vi "Run.vi"(0 "reg in":refnum<class "bronkhorst_reg_1.lvclass">, 1 "XB24 (F)":bool, 5 "SP":dbl caption="setpoint" step=0.01 format="%.2f", 7 "PV":dbl step=0.01 format="%.2f", 9 "PV_State":T5, 11 "error in (no error)":errorcluster, 12 "Y_in":dbl step=0.01 format="%.2f", 13 "Y_State":T5) -> (4 "reg out":refnum<class "bronkhorst_reg_1.lvclass">, 6 "Y_out":dbl format="%.2f", 8 "T":u32, 10 "End":bool, 15 "error out":errorcluster)   [LabVIEW 2019, in "bronkhorst_reg_1.lvclass"]
uses:
  bronkhorst_reg_1.lvclass
  Inputs/Ctl/Parameter State short.ctl
  ctl/Y_Lim_State.ctl
  ctl/ZY_control_short.ctl
  ctl/Z_State.ctl
  ctl/Y_state.ctl
  bronkhorst_reg_1.lvclass/bronkhorst_reg_1.ctl
  Inputs/Ctl/Sensor state.ctl
  Inputs/Ctl/Sensor alarm.ctl
  ctl/control param simple.ctl
  PID/PID Output Rate Limiter Ext.vi
  PID/PID Timing Estimation Ext.vi
  control.lvlib
  Inputs/Inputs.lvlib
panel:
  out "ZY_control":T1={"Start"=FALSE, "Z_HSw"=0, "Z_HSetState"=enum."on", "Y_HSw"=0, "Y_HSetState"=enum."hand", "SP"=0.0, "Y_H"=0.0, "Reset_ALR"=FALSE} {"Y_H" step=1.0; "SP" step=0.01 format="%.2f"}
  out "SpLim_State":T4=enum."increase"
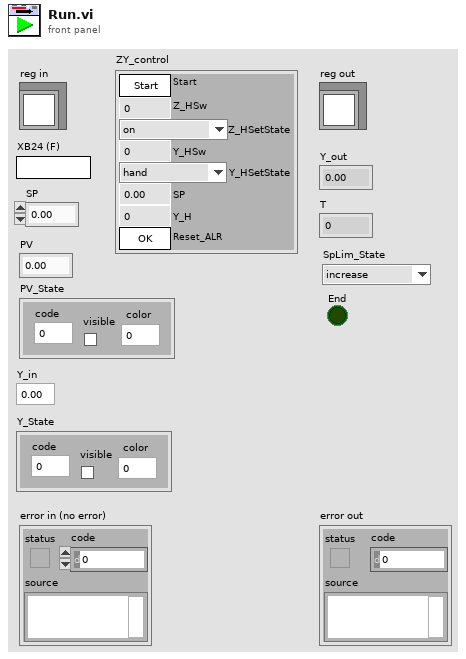
[diagram p1: front panel]
types:
  T1 = typedef "control.lvlib/ZY_control_short.ctl" = cluster{"Start":bool, "Z_HSw":u32, "Z_HSetState":T2, "Y_HSw":u32, "Y_HSetState":T3, "SP":dbl, "Y_H":dbl, "Reset_ALR":bool}
  T2 = typedef "control.lvlib/Z_State.ctl" = enum8{"initialization", "alarm", "disabled", "not ready", "stop ready", "reserv", "switched off", "reserv2", "switched on", "check", "on min", "decrease out", "on", "increase out", "on max"}
  T3 = typedef "control.lvlib/Y_state.ctl" = enum8{"initialize", "alarm", "min", "stop", "hand", "auto", "max"}
  T4 = typedef "control.lvlib/Y_Lim_State.ctl" = enum8{"initialization", "alarm", "stop", "decrease", "increase"}
  T5 = typedef "Inputs.lvlib/Parameter State short.ctl" = cluster{"code":i32, "visible":bool, "color":u32}
  T6 = typedef "Inputs.lvlib/Sensor state.ctl" = cluster{"source":string, "color":u32, "visible":bool}[]
  T7 = typedef "Inputs.lvlib/Sensor alarm.ctl" = cluster{"source":string, "color":u32, "visible":bool}[]
  T8 = typedef "control.lvlib/control param simple.ctl" = cluster{"output high":dbl, "alr value":dbl, "output low":dbl, "output time (t)":dbl}
  T9 = cluster{"Y_HSw":u32, "Y_HSetState":T3, "Y_ASetState":T3, "Y_DSetState":T3}
  T10 = typedef "control.lvlib/control param.ctl" = cluster{"proportional gain (Kc)":dbl, "integral time (Ti, s)":dbl, "derivative time (Td, s)":dbl, "output high":dbl, "output high start":dbl, "output high stop":dbl, "alr value":dbl, "output low":dbl, "output rate (EGU/s)":dbl, "setpoint max":dbl, "setpoint rate (EGU/min)":dbl, "stop rate (EGU/min)":dbl}
  T11 = typedef "control.lvlib/Y_source.ctl" = enum8{"initialize", "local disabled", "local hand", "hand", "auto", "dist"}
  T12 = enum8{"alarm", "min", "stop", "hand", "auto", "max"}
  T13 = typedef "control.lvlib/Y_Lim_ext_defs.ctl" = cluster{"reinitialize":bool, "SpLim_State":T4, "output":dbl, "Tick":u32, "output rate":dbl, "Y_Set":dbl, "Y_preSet":dbl}
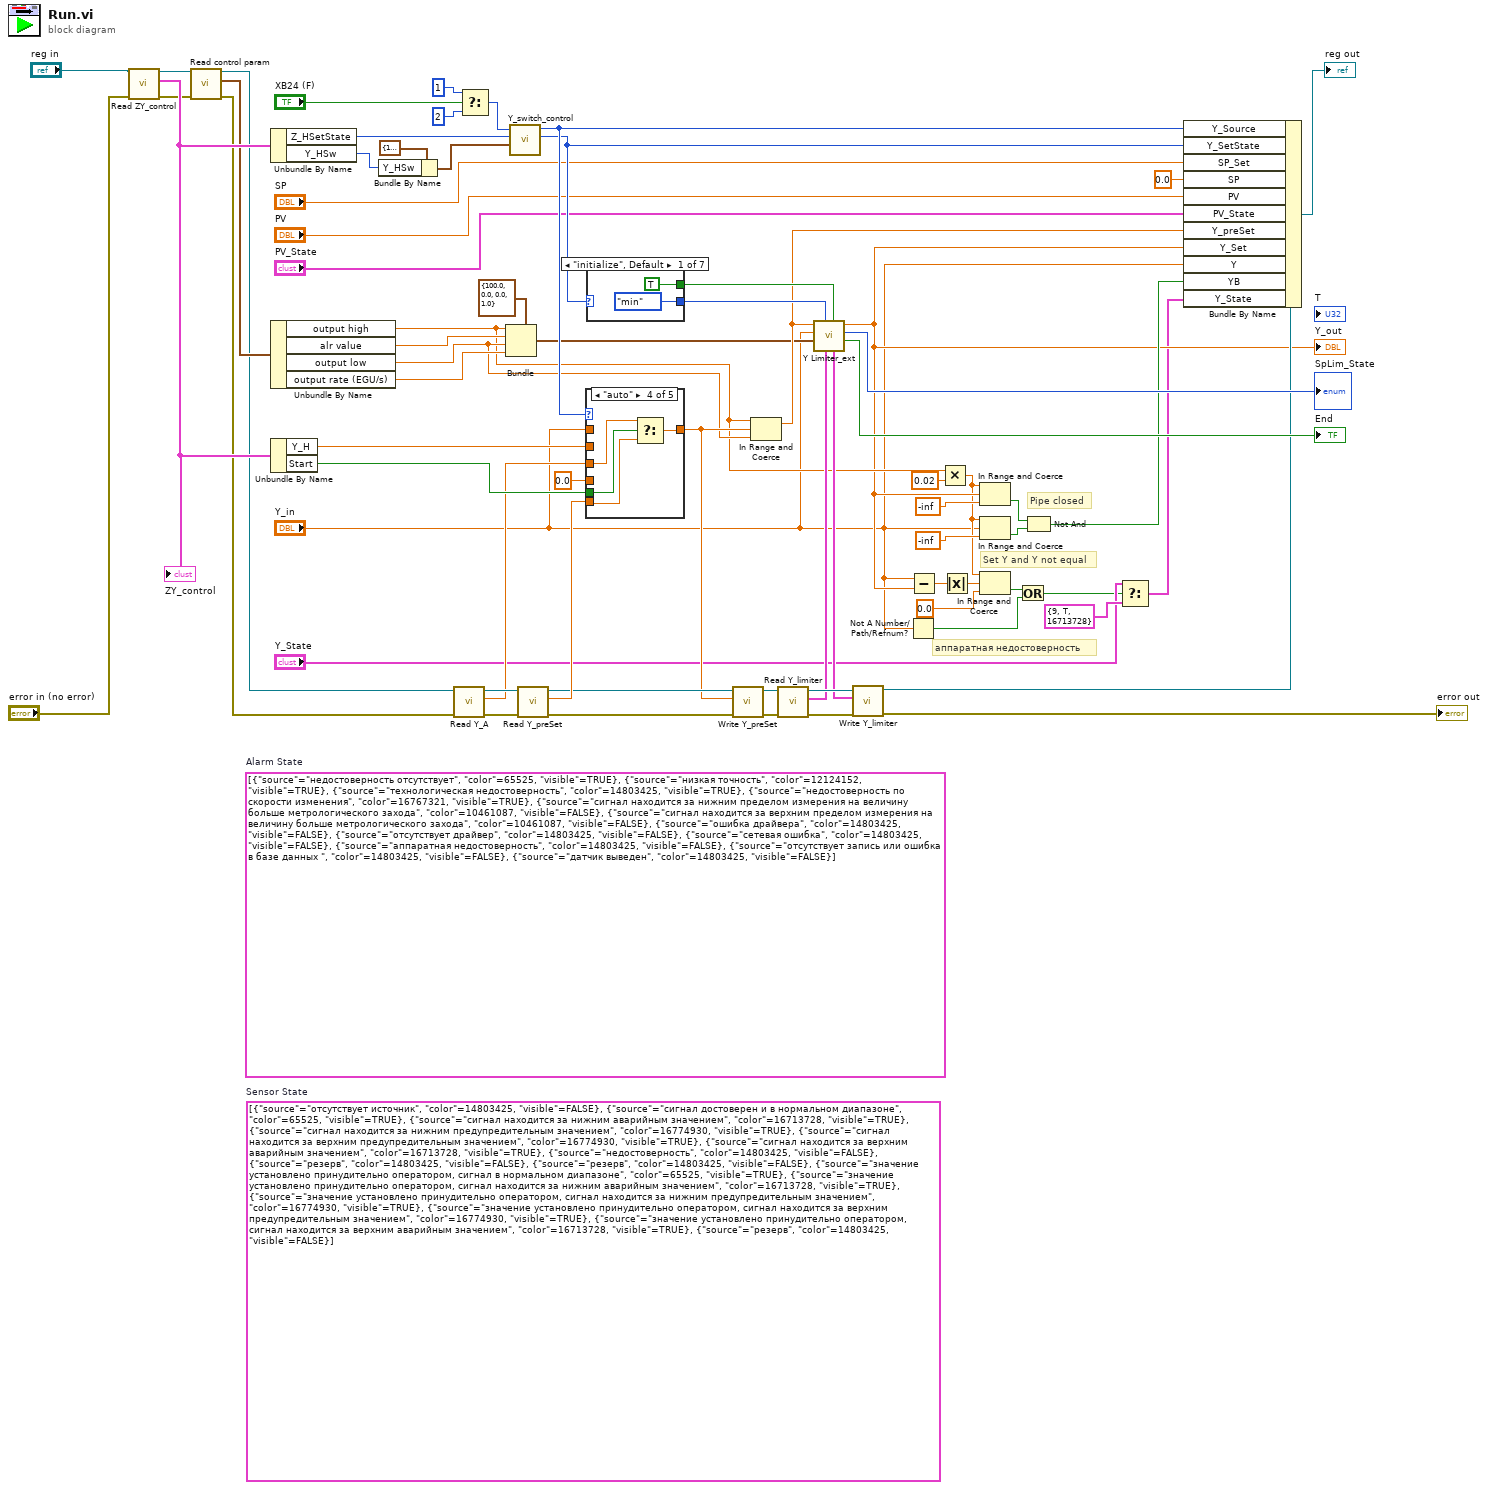
[diagram p0: block diagram]
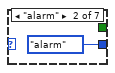
[diagram p2: hidden frame]
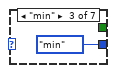
[diagram p3: hidden frame]
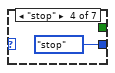
[diagram p4: hidden frame]
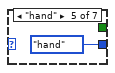
[diagram p5: hidden frame]
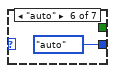
[diagram p6: hidden frame]
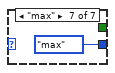
[diagram p7: hidden frame]
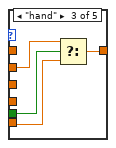
[diagram p10: hidden frame]
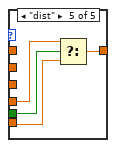
[diagram p11: hidden frame]
diagram:
  (unwired) T6 [{"source"="отсутствует источник", "color"=14803425, "visible"=FALSE}, {"source"="сигнал достоверен и в нормальном диапазоне", "color"=65525, "visible"=TRUE}, {"source"="сигнал находится за нижним аварийным значением", "color"=16713728, "visible"=TRUE}, {"source"="сигнал находится за нижним предупредительным значением", "color"=16774930, "visible"=TRUE}, {"source"="сигнал находится за верхним предупредительным значением", "color"=16774930, "visible"=TRUE}, {"source"="сигнал находится за верхним аварийным значением", "color"=16713728, "visible"=TRUE}, {"source"="недостоверность", "color"=14803425, "visible"=FALSE}, {"source"="резерв", "color"=14803425, "visible"=FALSE}, {"source"="резерв", "color"=14803425, "visible"=FALSE}, {"source"="значение установлено принудительно оператором, сигнал в нормальном диапазоне", "color"=65525, "visible"=TRUE}, {"source"="значение установлено принудительно оператором, сигнал находится за нижним аварийным значением", "color"=16713728, "visible"=TRUE}, {"source"="значение установлено принудительно оператором, сигнал находится за нижним предупредительным значением", "color"=16774930, "visible"=TRUE}, {"source"="значение установлено принудительно оператором, сигнал находится за верхним предупредительным значением", "color"=16774930, "visible"=TRUE}, {"source"="значение установлено принудительно оператором, сигнал находится за верхним аварийным значением", "color"=16713728, "visible"=TRUE}, {"source"="резерв", "color"=14803425, "visible"=FALSE}]  # Sensor State
  (unwired) T7 [{"source"="недостоверность отсутствует", "color"=65525, "visible"=TRUE}, {"source"="низкая точность", "color"=12124152, "visible"=TRUE}, {"source"="технологическая недостоверность", "color"=14803425, "visible"=TRUE}, {"source"="недостоверность по скорости изменения", "color"=16767321, "visible"=TRUE}, {"source"="сигнал находится за нижним пределом измерения на величину больше метрологического захода", "color"=10461087, "visible"=FALSE}, {"source"="сигнал находится за верхним пределом измерения на величину больше метрологического захода", "color"=10461087, "visible"=FALSE}, {"source"="ошибка драйвера", "color"=14803425, "visible"=FALSE}, {"source"="отсутствует драйвер", "color"=14803425, "visible"=FALSE}, {"source"="сетевая ошибка", "color"=14803425, "visible"=FALSE}, {"source"="аппаратная недостоверность", "color"=14803425, "visible"=FALSE}, {"source"="отсутствует запись или ошибка в базе данных ", "color"=14803425, "visible"=FALSE}, {"source"="датчик выведен", "color"=14803425, "visible"=FALSE}]  # Alarm State
  # "аппаратная недостоверность"
  # "Set Y and Y not equal"
  # "Pipe closed"
  n1 = call "Read ZY_control.vi"("error in (no error)"="error in (no error)", "reg in"="reg in") -> ("error out"=w31:errorcluster, "ZY_control"=w35:T1, "reg out"=w32:refnum<class "bronkhorst_reg_1.lvclass">)  [unwired: 7 in]
  "ZY_control" <- w35
  n2 = call "Read control param.vi"("error in (no error)"=w31, "reg in"=w32) -> ("error out"=w23:errorcluster, "control param"=w30:T10, "reg out"=w24:refnum<class "bronkhorst_reg_1.lvclass">)  [unwired: 7 in]
  n3 = Unbundle By Name(w35) -> ("Z_HSetState"=w39:T2, "Y_HSw"=w42:u32)
  n4 = Unbundle By Name(w30) -> ("output high"=w18:dbl, "alr value"=w27:dbl, "output low"=w25:dbl, "output rate (EGU/s)"=w26:dbl)
  n5 = Unbundle By Name(w35) -> ("Y_H"=w33:dbl, "Start"=w34:bool)
  n6 = Bundle By Name(cluster=T9 {"Y_HSw"=1, "Y_HSetState"=enum."hand", "Y_ASetState"=enum."hand", "Y_DSetState"=enum."auto"} ("Y_Set"), "Y_HSw"=w42) -> (w38:T9)
  n7 = call "Read Y_A.vi"("error in (no error)"=w23, "reg in"=w24) -> ("error out"=w21:errorcluster, "Y_A"=w20:dbl, "reg out"=w22:refnum<class "bronkhorst_reg_1.lvclass">)  [unwired: 7 in]
  n8 = Select(t=u32 1, s="XB24 (F)", f=u32 2 ("Y_HSw")) -> (s? t:f=w68:u32)
  n9 = Bundle(cluster=T8 {"output high"=100.0, "alr value"=0.0, "output low"=0.0, "output time (t)"=1.0} ("control param"), "output high"=w18, "alr value"=w27, "output low"=w25, "output time (t)"=w26) -> (w28:T8)
  n10 = call "Y_switch_control.vi"("Y"=w38, "Z_State"=w39, "Y_LSw (2-auto)"=w68) -> ("Y_SetState"=w65:T3, "Y_Source"=w66:T11)  [unwired: 7 in]
  n11 = call "Read Y_preSet.vi"("error in (no error)"=w21, "reg in"=w22) -> ("error out"=w50:errorcluster, "Y_preSet"=w55:dbl, "reg out"=w54:refnum<class "bronkhorst_reg_1.lvclass">)  [unwired: 7 in]
  n12 = case shown="\"auto\"" w66 {
    tunnel: w33 -> [_ _ w73 _ _]
    tunnel: "Y_in" -> [w71 w72 _ _ _]
    tunnel: 0.0 ("Y_A") -> [_ _ _ _ w83]
    tunnel: [w71 w72 w76 w80 w84] -> w53
    tunnel: w20 -> [_ _ _ w77 _]
    tunnel: w55 -> [_ _ w75 w79 w82]
    tunnel: w34 -> [_ _ w74 w78 w81]
    frame "local disabled", Default {
    }
    frame "local hand" {
    }
    frame "hand" {
      n13 = Select(t=w73, s=w74, f=w75) -> (s? t:f=w76:dbl)
    }
    frame "auto" {
      n14 = Select(t=w77, s=w78, f=w79) -> (s? t:f=w80:dbl)
    }
    frame "dist" {
      n15 = Select(t=w83, s=w81, f=w82) -> (s? t:f=w84:dbl)
    }
  }
  n16 = case shown="\"initialize\", Default" w65 {
    tunnel: [T12."min" ("X1(SetState)") T12."alarm" ("X1(SetState)") T12."min" ("X1(SetState)") T12."stop" ("X1(SetState)") T12."hand" ("X1(SetState)") T12."auto" ("X1(SetState)") T12."max" ("X1(SetState)")] -> w60
    tunnel: [TRUE _ _ _ _ _ _] -> w61
    frame "initialize", Default {
    }
    frame "alarm" {
    }
    frame "min" {
    }
    frame "stop" {
    }
    frame "hand" {
    }
    frame "auto" {
    }
    frame "max" {
    }
  }
  n17 = call "Write Y_preSet.vi"("error in (no error)"=w50, "Y_preSet"=w53, "reg in"=w54) -> ("error out"=w51:errorcluster, "reg out"=w52:refnum<class "bronkhorst_reg_1.lvclass">)  [unwired: 7 in]
  n18 = In Range and Coerce(upper limit=w18, x=w53, lower limit=w25) -> (coerced(x)=w56:dbl)  [unwired: 1 out]
  n19 = call "Read Y_limiter.vi"("error in (no error)"=w51, "reg in"=w52) -> ("error out"=w47:errorcluster, "Y_limiter"=w48:T13, "reg out"=w49:refnum<class "bronkhorst_reg_1.lvclass">)  [unwired: 7 in]
  n20 = call "Y Limiter_ext.vi"("reinitialize? (F)"=w61, "Y_limiter_old"=w48, "X1(SetState)"=w60, "Y param"=w28, "Y (NaN)"="Y_in", "Y_Set"=w56) -> ("End"=→"End":bool, "SpLim_State"=→"SpLim_State":T4, "output"=w12:dbl, "Y_limiter"=w46:T13)  [unwired: 2 in]
  "Y_out" <- w12
  n21 = call "Write Y_limiter.vi"("error in (no error)"=w47, "Y_limiter"=w46, "reg in"=w49) -> ("error out"=→"error out":errorcluster, "reg out"=w45:refnum<class "bronkhorst_reg_1.lvclass">)  [unwired: 7 in]
  n22 = Not A Number/Path/Refnum?(number/path/refnum="Y_in") -> (NaN/Path/Refnum?=w2:bool)
  n23 = Subtract(x="Y_in", y=w12) -> (x-y=w10:dbl)
  n24 = Multiply(x=w18, y=0.02) -> (x*y=w11:dbl)
  n25 = Absolute Value(x=w10) -> (abs(x)=w8:dbl)
  n26 = In Range and Coerce(upper limit=w11, x=w12, lower limit=-inf) -> (In Range?=w15:bool)  [unwired: 1 out]
  n27 = In Range and Coerce(upper limit=w11, x="Y_in", lower limit=-inf) -> (In Range?=w14:bool)  [unwired: 1 out]
  n28 = In Range and Coerce(upper limit=w11, x=w8, lower limit=0.0) -> (In Range?=w7:bool)  [unwired: 1 out]
  n29 = Or(x=w7, y=w2) -> (x .or. y?=w3:bool)
  n30 = Not And(1:w14, 2:w15) -> (0:w13:bool)
  n31 = Select(t="Y_State", s=w3, f=cluster{"code":i32, "visible":bool, "color":u32} {"code"=9, "visible"=TRUE, "color"=16713728}) -> (s? t:f=w1:T5)
  n32 = Bundle By Name(cluster=w45, "Y_Source"=w66, "Y_SetState"=w65, "SP_Set"="SP", "SP"=0.0, "PV"="PV", "PV_State"="PV_State", "Y_preSet"=w56, "Y_Set"=w12, "Y"="Y_in", "YB"=w13, "Y_State"=w1) -> (→"reg out":refnum<class "bronkhorst_reg_1.lvclass">)
